vi "RemovesZeros.vi"(1 "5.3.1 MissionTimeAuto 2":dbl) -> (0 "5.3.1 MissionTimeAuto":dbl)   [LabVIEW 2010]
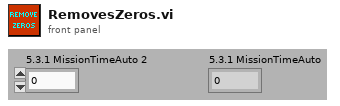
[diagram p1: front panel]
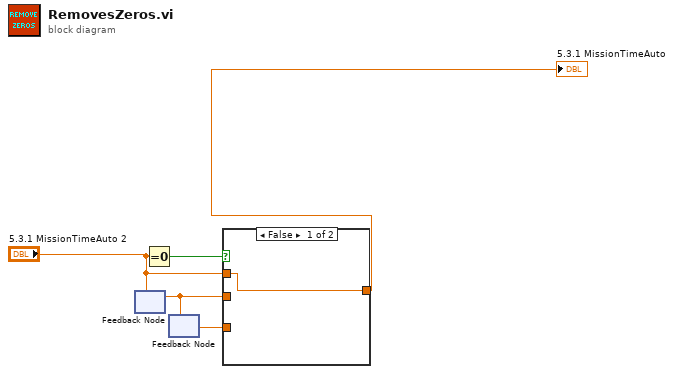
[diagram p0: block diagram]
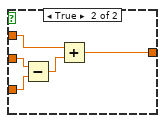
[diagram p2: hidden frame]
diagram:
  n1 = feedback #1() -> (w2:dbl)  [unwired: 1 in]
  n2 = feedback-in #1("5.3.1 MissionTimeAuto 2") -> ()
  n3 = Equal To 0?(x="5.3.1 MissionTimeAuto 2") -> (x = 0?=w1:bool)
  n4 = feedback #2() -> (w3:dbl)  [unwired: 1 in]
  n5 = feedback-in #2(w2) -> ()
  n6 = case shown="False" w1 {
    tunnel: w2 -> [_ w11]
    tunnel: w3 -> [_ w10]
    tunnel: "5.3.1 MissionTimeAuto 2" -> [w6 w9]
    tunnel: [w6 w7] -> w5
    frame False {
    }
    frame True {
      n7 = Subtract(x=w11, y=w10) -> (x-y=w8:dbl)
      n8 = Add(x=w9, y=w8) -> (x+y=w7:dbl)
    }
  }
  "5.3.1 MissionTimeAuto" <- w5
